vi "comm close2.vi"(4 "error in (no error)":errorcluster, 6 "close all? (F)":bool, 7 "Comm Handle":u32) -> (0 "error out":errorcluster)   [LabVIEW 2013, in "lvserial.lvlib"]
doc: "Closes the serial port."
uses:
  lvserial.lvlib
  lvserial.dll
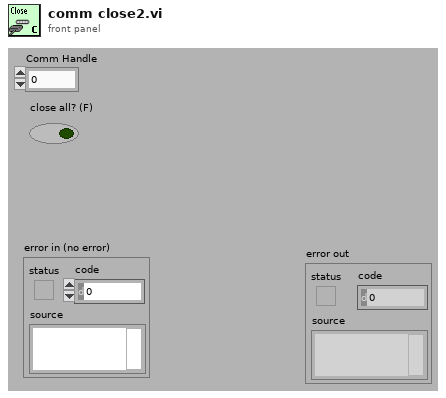
[diagram p1: front panel]
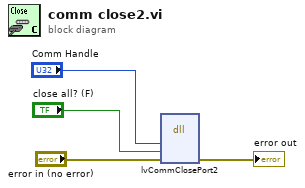
[diagram p0: block diagram]
diagram:
  n1 = dll-call lib="lvserial.dll" fn="lvCommClosePort2"("hComm"="Comm Handle", "close all? (F)"="close all? (F)", "error in (no error)"="error in (no error)") -> ("error in (no error)"=→"error out":errorcluster)  [unwired: 5 in, 3 out]
